vi "Handle_Error.vi"(8 "error in (no error)":errorcluster, 10 "Variant":variant) -> (0 "error out":errorcluster)   [LabVIEW 2020, in "Error handler.lvlib"]
doc: "Send Handle Error Message to the Queue."
uses:
  Error handler.lvlib
  Private Controls/Message Cluster.ctl
  Private Controls/Message enum.ctl
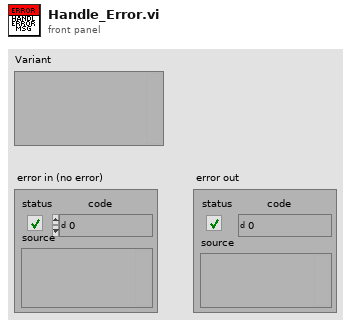
[diagram p1: front panel]
types:
  T1 = typedef "Error handler.lvlib/Message Cluster.ctl" = cluster{"Message":T2, "Data":variant}
  T2 = typedef "Error handler.lvlib/Message enum.ctl" = enum16{"Initialize", "State", "Error", "Exit", "Log", "Process_Sensor_Error", "Display_Console_Error", "User_Console_Error"}
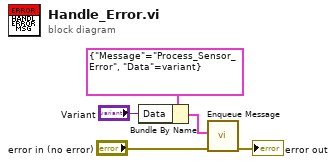
[diagram p0: block diagram]
diagram:
  n1 = Bundle By Name(cluster=T1 {"Message"=enum."Process_Sensor_Error", "Data"=variant} ("Message Cluster"), "Data"="Variant") -> (w1:T1)
  n2 = call "Enqueue Message.vi"("error in (no error)"="error in (no error)", "Element"=w1) -> ("error out"=→"error out":errorcluster)  [unwired: 9 in]
